vi "Sort Types.vi"(10 "Types in":T1[](array[typedef])) -> (2 "Types":T1[](array[typedef]))   [LabVIEW 2022 SP3, in "FlexBlocks Support.lvlib"]
uses:
  FlexBlocks Support.lvlib
  Type Descriptor.ctl
  Terminal Direction.ctl
  Value Mode.ctl
  Special Terminal.ctl
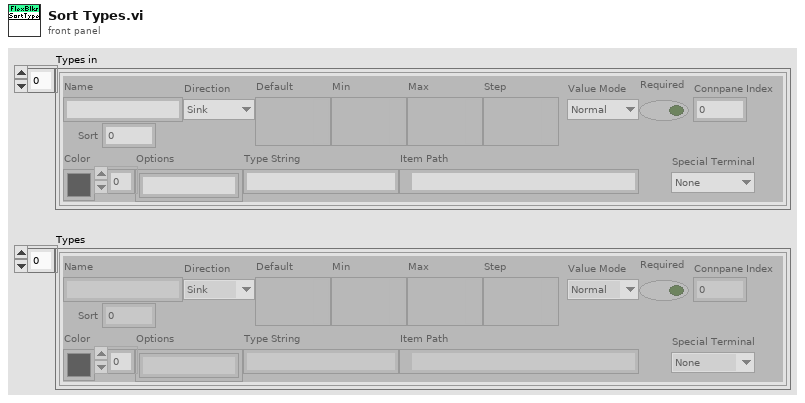
[diagram p1: front panel]
types:
  T1 = typedef "FlexBlocks Support.lvlib/Type Descriptor.ctl" = cluster{"Name":string, "Direction":T2, "Default":variant, "Min":variant, "Max":variant, "Step":variant, "Value Mode":T3, "Color":u32, "Options":string[], "Type String":string, "Item Path":path, "Required":bool, "Connpane Index":i32, "Special Terminal":T4, "Sort":i32}
  T2 = typedef "FlexBlocks Support.lvlib/Terminal Direction.ctl" = enum16{"Sink", "Source"}
  T3 = typedef "FlexBlocks Support.lvlib/Value Mode.ctl" = enum16{"Normal", "Range", "Select"}
  T4 = typedef "FlexBlocks Support.lvlib/Special Terminal.ctl" = enum16{"None", "Action", "Init", "Tag", "State in", "State out", "Error"}
  T5 = cluster{i32, "Name":string, "Type Descriptor":T1}
  T6 = cluster{i32, "Name":string, "Type Descriptor":T1}[]
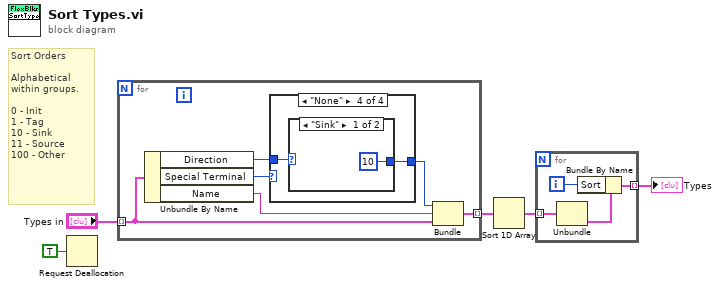
[diagram p0: block diagram]
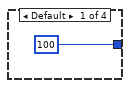
[diagram p2: hidden frame]
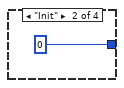
[diagram p3: hidden frame]
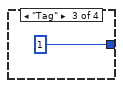
[diagram p4: hidden frame]
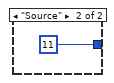
[diagram p5: hidden frame]
diagram:
  # "Sort Orders\n\nAlphabetical within groups.\n\n0 - Init\n1 - Tag\n10 - Sink\n11 - Source\n100 - Other"
  n1 = Request Deallocation(TRUE ("flag")) -> ()
  n2 = for {
    tunnel: "Types in" -> [w7] mode=indexing
    tunnel: [w6] -> w3 mode=indexing
    n3 = Unbundle By Name(w7) -> ("Direction"=w10:T2, "Special Terminal"=w11:T4, "Name"=w8:string)
    n4 = case shown="\"None\"" w11 {
      tunnel: w10 -> [_ _ _ w16]
      tunnel: [100 0 1 w15] -> w9
      frame Default {
      }
      frame "Init" {
      }
      frame "Tag" {
      }
      frame "None" {
        n5 = case shown="\"Sink\"" w16 {
          tunnel: [10 11] -> w15
          frame "Sink" {
          }
          frame "Source" {
          }
        }
      }
    }
    n6 = Bundle(w9, "Name"=w8, "Type Descriptor"=w7) -> (w6:T5)  [unwired: 1 in]
  }
  n7 = Sort 1D Array(array=w3) -> (sorted array=w2:T6)
  n8 = for {
    tunnel: w2 -> [w22] mode=indexing
    tunnel: [w19] -> w1 mode=indexing
    i -> [w20]
    n9 = Unbundle(w22) -> ("Type Descriptor"=w21:T1)  [unwired: 2 out]
    n10 = Bundle By Name(cluster=w21, "Sort"=w20) -> (w19:T1)
  }
  "Types" <- w1
